vi "4461 - Create AO waveforms.vi"(6 "time delay":dbl, 8 "error in (no error)":errorcluster, 9 "sampling info":cluster{"Fs":dbl, "#s":i32}={"Fs"=1000.0, "#s"=1000} {"Fs" format="%.2p"}, 10 "reset signal":bool, 11 "AO":T1={"AO amp (V)"=[0.1, 0.09, 0.08, 0.07, 0.06, 0.05, 0.04, 0.03], "AO DC (V)"=[0.0, 0.0, 0.0, 0.0, 0.0, 0.0, 0.0, 0.0], "AO f (Hz)"=[13.0, 13.0, 13.0, 13.0, 13.0, 13.0, 13.0, 13.0], "AO phi (deg)"=[0.0, 0.0, 0.0, 0.0, 0.0, 0.0, 0.0, 0.0], "function"=[enum."Sine Wave", enum."Sine Wave", enum."Sine Wave", enum."Sine Wave", enum."Sine Wave", enum."Sine Wave", enum."Sine Wave", enum."Sine Wave"]} {"AO f (Hz)" min=0.001 max=10000.0; "AO DC (V)" format="%#_6p"; "AO amp (V)" format="%#_6p"}) -> (0 "error out":errorcluster, 1 "phase out":dbl[](array[numeric]), 2 "AO Array":waveform(dbl)[](array[waveform]), 3 "AO 2":T1={"AO amp (V)"=[0.1, 0.09, 0.08, 0.07, 0.06, 0.05, 0.04, 0.03], "AO DC (V)"=[0.0, 0.0, 0.0, 0.0, 0.0, 0.0, 0.0, 0.0], "AO f (Hz)"=[13.0, 13.0, 13.0, 13.0, 13.0, 13.0, 13.0, 13.0], "AO phi (deg)"=[0.0, 0.0, 0.0, 0.0, 0.0, 0.0, 0.0, 0.0], "function"=[enum."Sine Wave", enum."Sine Wave", enum."Sine Wave", enum."Sine Wave", enum."Sine Wave", enum."Sine Wave", enum."Sine Wave", enum."Sine Wave"]} {"AO f (Hz)" min=0.001 max=10000.0; "AO DC (V)" format="%#_6p"; "AO amp (V)" format="%#_6p"})   [LabVIEW 2020]
uses:
  Typedefs/AO-cluster.ctl
  Typedefs/AO_Amp-array.ctl
  Typedefs/AO_DC-array.ctl
  Typedefs/AO_f-array.ctl
  Typedefs/AO_phi-array.ctl
  Typedefs/Function-array.ctl
  Typedefs/Function-enum.ctl
  <vilib>/measure/NI_MABase.lvlib
panel:
  out "Waveform Chart":dbl[][](graph)
  out "Waveform Graph 2":waveform(dbl)[](graph)
  out "Numeric":i32
  # "0"
  # "1"
  # "2"
  # "3"
  # "4"
  # "5"
  # "6"
  # "7"
  # "0"
  # "1"
  # "2"
  # "3"
  # "4"
  # "5"
  # "6"
  # "7"
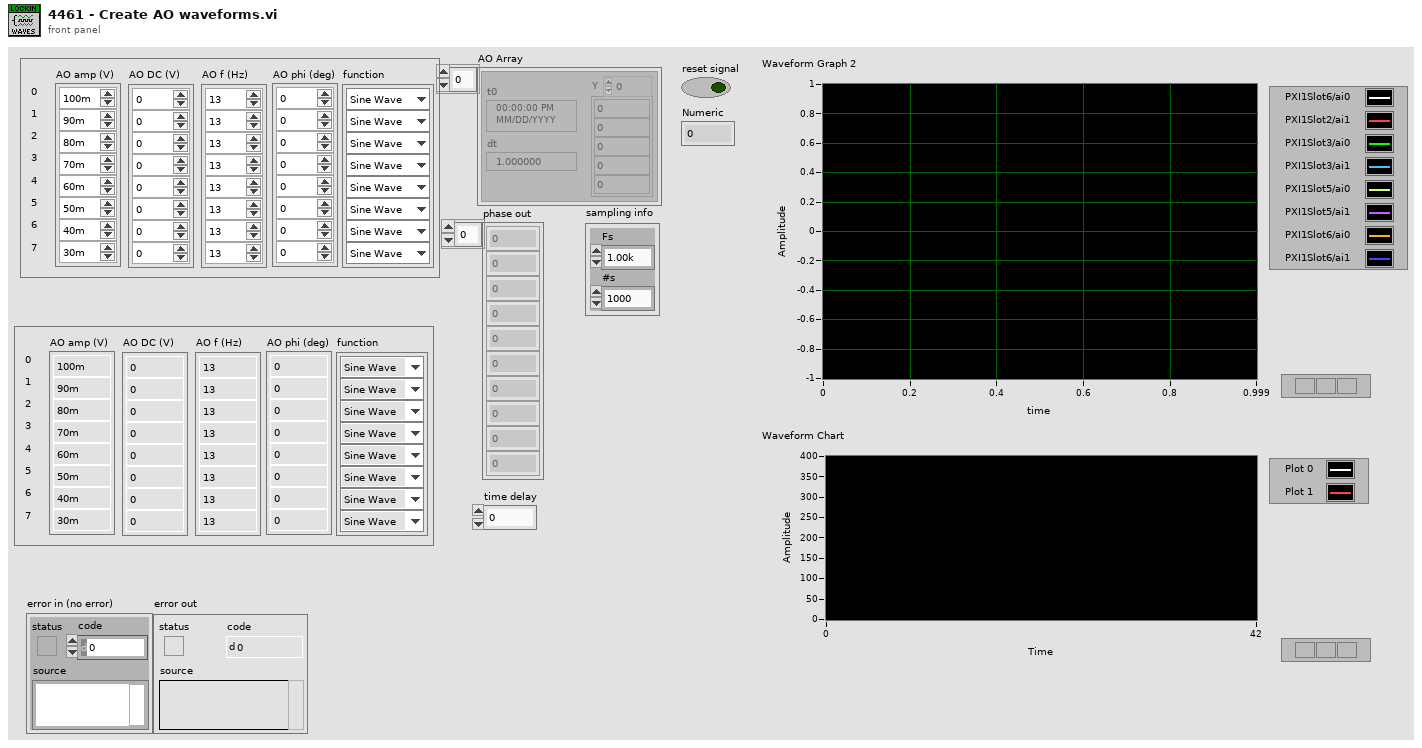
[diagram p1: front panel]
types:
  T1 = typedef "AO-cluster.ctl" = cluster{"AO amp (V)":T2, "AO DC (V)":T3, "AO f (Hz)":T4, "AO phi (deg)":T5, "function":T6}
  T2 = typedef "AO_Amp-array.ctl" = dbl[]
  T3 = typedef "AO_DC-array.ctl" = dbl[]
  T4 = typedef "AO_f-array.ctl" = dbl[]
  T5 = typedef "AO_phi-array.ctl" = dbl[]
  T6 = typedef "Function-array.ctl" = T7[]
  T7 = typedef "Function-enum.ctl" = enum16{"Sine Wave", "Triangle Wave", "Square Wave", "Sawtooth Wave"}
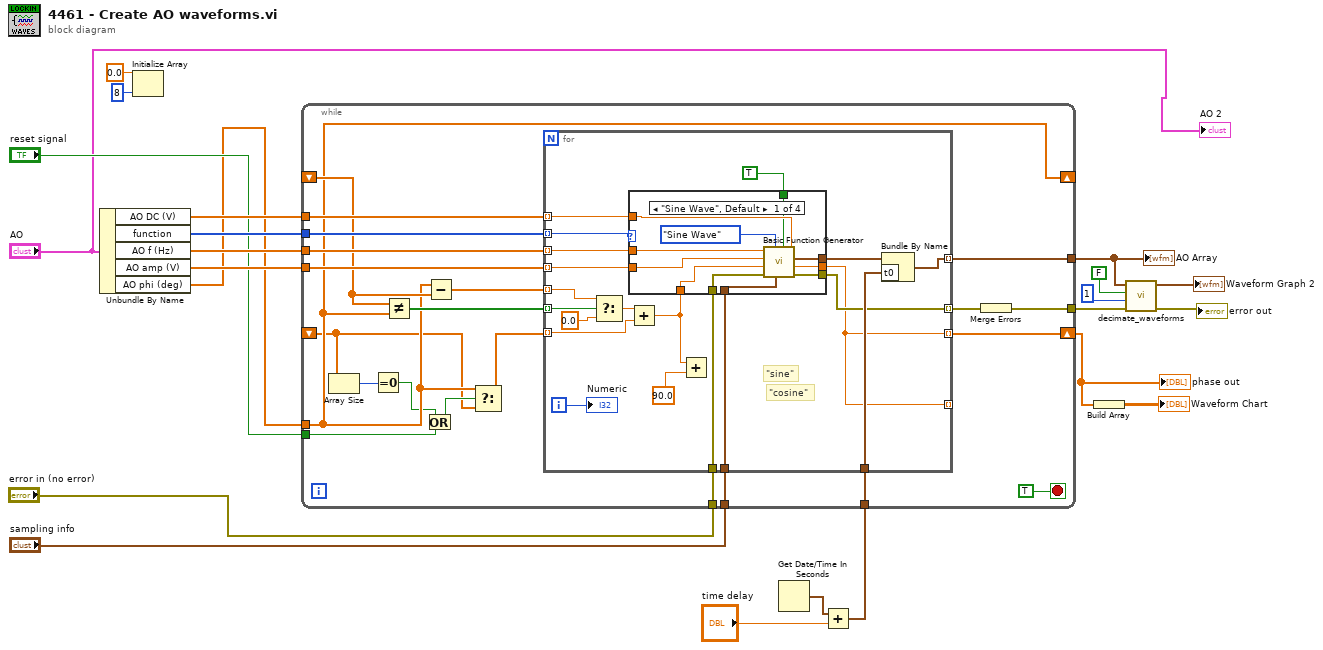
[diagram p0: block diagram]
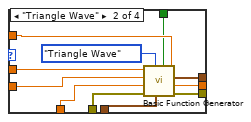
[diagram p2: hidden frame]
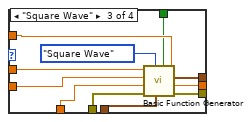
[diagram p3: hidden frame]
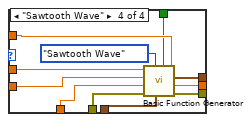
[diagram p4: hidden frame]
diagram:
  n1 = Unbundle By Name("AO") -> ("AO DC (V)"=w21:T3, "function"=w22:T6, "AO f (Hz)"=w18:T4, "AO amp (V)"=w19:T2, "AO phi (deg)"=w2:T5)
  n2 = Initialize Array(0.0 ("element"), 8 ("dimension size")) -> ()  [unwired: 1 out]
  n3 = Get Date/Time In Seconds() -> (seconds since 1Jan1904=w9:timestamp)
  n4 = Add(x=w9, y="time delay") -> (x+y=w7:timestamp)
  n5 = while {
    tunnel: w22 -> [w44]
    tunnel: w21 -> [w43]
    tunnel: "sampling info" -> [w42]
    tunnel: [w41] -> w14
    tunnel: w19 -> [w40]
    tunnel: w2 -> [w31]
    tunnel: w18 -> [w39]
    shift-right: [w31] -> _
    shift-left: _ -> [w36]
    shift-right: [w34] -> w5
    shift-left: _ -> [w23]
    tunnel: w7 -> [w33]
    tunnel: "reset signal" -> [w28]
    tunnel: "error in (no error)" -> [w26]
    tunnel: [w24] -> w11
    stop <- TRUE stop-if-true
    n6 = Array Size(array=w23) -> (size(s)=w32:i32)
    n7 = Equal To 0?(x=w32) -> (x = 0?=w29:bool)
    n8 = Not Equal?(x=w36, y=w31) -> (x != y?=w37:bool[])
    n9 = Or(x=w29, y=w28) -> (x .or. y?=w30:bool)
    n10 = Subtract(x=w31, y=w36) -> (x-y=w35:T5)
    n11 = Select(t=w31, s=w30, f=w23) -> (s? t:f=w27:T5)
    n12 = for {
      tunnel: w44 -> [w45] mode=indexing
      tunnel: w39 -> [w64] mode=indexing
      tunnel: w40 -> [w48] mode=indexing
      tunnel: w43 -> [w63] mode=indexing
      tunnel: [w53] -> w41 mode=indexing
      tunnel: w42 -> [w46]
      tunnel: w37 -> [w57] mode=indexing
      tunnel: w35 -> [w59] mode=indexing
      tunnel: [w50] -> w34 mode=indexing
      tunnel: w27 -> [w49] mode=indexing
      tunnel: w33 -> [w56]
      tunnel: [w50] -> _ mode=indexing
      tunnel: w26 -> [w52]
      tunnel: [w51] -> w25 mode=indexing
      i -> [w55]
      # "\"cosine\""
      # "\"sine\""
      n13 = Select(t=w59, s=w57, f=0.0) -> (s? t:f=w60:dbl)
      n14 = Add(x=w60, y=w49) -> (x+y=w47:dbl)
      n15 = case shown="\"Sine Wave\", Default" w45 {
        tunnel: w64 -> [w75 w86 w97 w108]
        tunnel: w63 -> [w74 w85 w96 w107]
        tunnel: [w73 w84 w95 w106] -> w62
        tunnel: TRUE ("reset signal") -> [w72 w83 w94 w105]
        tunnel: w52 -> [w71 w82 w93 w104]
        tunnel: [w70 w81 w92 w103] -> w51
        tunnel: [w69 w80 w91 w102] -> w50
        tunnel: w48 -> [w68 w79 w90 w101]
        tunnel: w47 -> [w67 w78 w89 w100]
        tunnel: w46 -> [w66 w77 w88 w99]
        frame "Sine Wave", Default {
          n16 = call <vilib>:"Basic Function Generator.vi"("offset"=w74, "reset signal"=w72, "sampling info"=w66, "signal type"=Function-enum."Sine Wave" ("Signal Type"), "error in (no error)"=w71, "phase"=w67, "amplitude"=w68, "frequency"=w75) -> ("error out"=w70:errorcluster, "phase out"=w69:dbl, "signal out"=w73:waveform(dbl))  [unwired: 1 in]
        }
        frame "Triangle Wave" {
          n17 = call <vilib>:"Basic Function Generator.vi"("offset"=w85, "reset signal"=w83, "sampling info"=w77, "signal type"=Function-enum."Triangle Wave" ("Signal Type"), "error in (no error)"=w82, "phase"=w78, "amplitude"=w79, "frequency"=w86) -> ("error out"=w81:errorcluster, "phase out"=w80:dbl, "signal out"=w84:waveform(dbl))  [unwired: 1 in]
        }
        frame "Square Wave" {
          n18 = call <vilib>:"Basic Function Generator.vi"("offset"=w96, "reset signal"=w94, "sampling info"=w88, "signal type"=Function-enum."Square Wave" ("Signal Type"), "error in (no error)"=w93, "phase"=w89, "amplitude"=w90, "frequency"=w97) -> ("error out"=w92:errorcluster, "phase out"=w91:dbl, "signal out"=w95:waveform(dbl))  [unwired: 1 in]
        }
        frame "Sawtooth Wave" {
          n19 = call <vilib>:"Basic Function Generator.vi"("offset"=w107, "reset signal"=w105, "sampling info"=w99, "signal type"=Function-enum."Sawtooth Wave" ("Signal Type"), "error in (no error)"=w104, "phase"=w100, "amplitude"=w101, "frequency"=w108) -> ("error out"=w103:errorcluster, "phase out"=w102:dbl, "signal out"=w106:waveform(dbl))  [unwired: 1 in]
        }
      }
      n20 = Add(x=w47, y=90.0) -> ()  [unwired: 1 out]
      n21 = Bundle By Name(cluster=w62, "t0"=w56) -> (w53:waveform(dbl))
      "Numeric" <- w55
    }
    n22 = Merge Errors(w25) -> (w24:errorcluster)
  }
  "AO Array" <- w14
  "phase out" <- w5
  n23 = Build Array(w5) -> (→"Waveform Chart":dbl[][])
  n24 = call "decimate_waveforms.vi"("Input Signal"=w14, "averaging"=FALSE, "decimating factor"=1, "error in (no error)"=w11) -> ("Decimated Waveforms"=→"Waveform Graph 2":waveform(dbl)[], "error out"=→"error out":errorcluster)  [unwired: 5 in]
  "AO 2" <- "AO"
